vi "replay voltage scaling calculation.vi"(7 "max ao voltage":dbl, 8 "maximum voltage":dbl=10.0, 9 "maximum speed (RPM)":dbl=10000.0, 10 "threshold voltage":dbl, 11 "threshold speed (RPM)":dbl) -> (2 "intercept (b)":fxp<+/-,18,3>, 3 "slope (m)":fxp<+,18,6>)   [LabVIEW 2013]
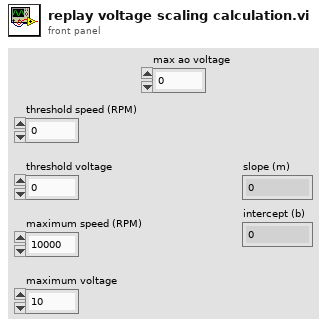
[diagram p1: front panel]
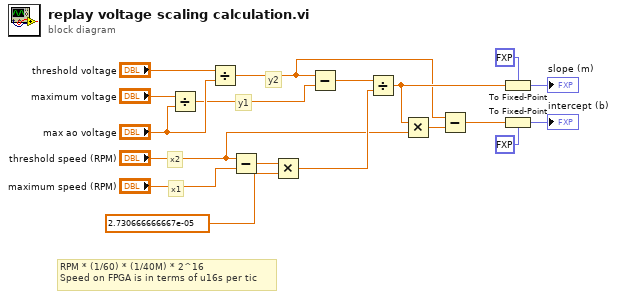
[diagram p0: block diagram]
diagram:
  # "x1"
  # "x2"
  # "y2"
  # "y1"
  # "RPM * (1/60) * (1/40M) * 2^16\nSpeed on FPGA is in terms of u16s per tic"
  n1 = Divide(x="maximum voltage", y="max ao voltage") -> (x/y=w11:dbl)
  n2 = Divide(x="threshold voltage", y="max ao voltage") -> (x/y=w2:dbl)
  n3 = Subtract(x="threshold speed (RPM)", y="maximum speed (RPM)") -> (x-y=w8:dbl)
  n4 = Multiply(x=w8, y=2.730666666667e-05) -> (x*y=w7:dbl)
  n5 = Subtract(x=w2, y=w11) -> (x-y=w10:dbl)
  n6 = Divide(x=w10, y=w7) -> (x/y=w4:dbl)
  n7 = Multiply(x=w4, y="threshold speed (RPM)") -> (x*y=w3:dbl)
  n8 = Subtract(x=w2, y=w3) -> (x-y=w1:dbl)
  n9 = To Fixed-Point(fixed-point type=fxp<+,18,6> 0.0, number=w4) -> (fixed-point=→"slope (m)":fxp<+,18,6>)
  n10 = To Fixed-Point(fixed-point type=fxp<+/-,18,3> 0.0, number=w1) -> (fixed-point=→"intercept (b)":fxp<+/-,18,3>)
